vi "GT Add Watch Var.vi"(8 "error in (no error)":errorcluster caption="错误输入（无错误）", 10 "pVar":cluster{"type":u16, "index":u16, "id":u16}, 11 "cardNum":i16) -> (0 "error out":errorcluster caption="错误输出", 3 "function return":i16)   [LabVIEW 2020, in "gts1.lvlib"]
doc: "GT_API GT_AddWatchVar(short cardNum,const TWatchVar *pVar);"
uses:
  gts1.lvlib
  dll/32bit/multi_card/gts.dll
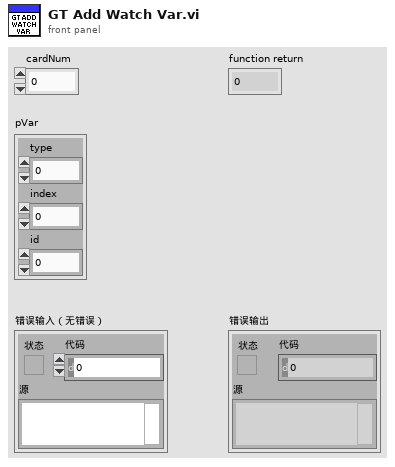
[diagram p1: front panel]
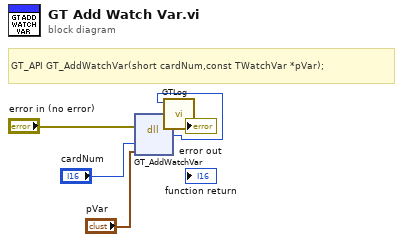
[diagram p0: block diagram]
diagram:
  # "GT_API GT_AddWatchVar(short cardNum,const TWatchVar *pVar);"
  n1 = dll-call lib="C:/1228/dll/32bit/multi_card/gts.dll" fn="GT_AddWatchVar"(error in="error in (no error)", "cardNum"="cardNum", "pVar"="pVar") -> (error out=w3:errorcluster, "return type"=w1:i16)  [unwired: 4 in, 1 out]
  n2 = call "GTLog.vi"("error in (no error)"=w3, "Numeric"=w1) -> ("error out"=→"error out":errorcluster)  [unwired: 9 in]
